vi "Is Command or Response.vi"(8 "error in (no error)":errorcluster, 11 "Command/Response Refnum in":T1 format="%.0x") -> (0 "error out":errorcluster, 2 "Is Command?":bool, 3 "Command/Response out":string)   [LabVIEW 2018, in "Instrument Addon Scripting API.lvlib"]
uses:
  Instrument Addon Scripting API.lvlib
  <vilib>/NI Veristand/Custom Device API/Custom Device Item Ref.ctl
  Addon/Addon Shared/SubVIs/Constants.vi
  Addon/Addon Shared/Instrument Addon Shared.lvlib
  <vilib>/NI VeriStand/Custom Device API/Custom Device API.lvlib
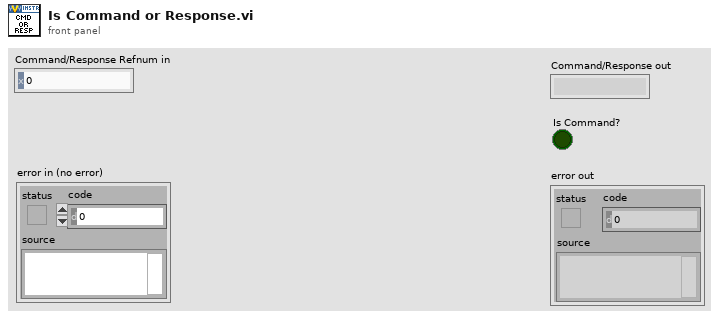
[diagram p1: front panel]
types:
  T1 = typedef "Custom Device API.lvlib/Custom Device Item Ref.ctl" = u64
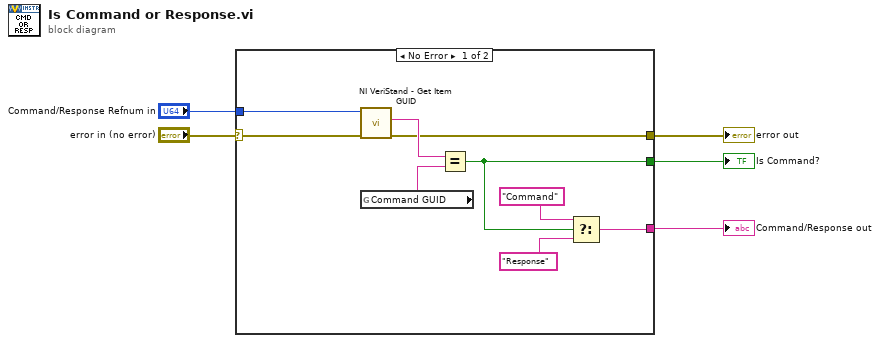
[diagram p0: block diagram]
diagram:
  n1 = case shown="No Error" "error in (no error)" {
    selector: "error in (no error)" -> [w6 w15]
    tunnel: [w14 _] -> w5
    tunnel: [w11 w15] -> w4
    tunnel: "Command/Response Refnum in" -> [w8 _]
    tunnel: [w7 _] -> w2
    frame No Error {
      n2 = call <vilib>:"NI VeriStand - Get Item GUID.vi"("error in (no error)"=w6, "Item Ref in"=w8) -> ("error out"=w11:errorcluster, "GUID"=w12:string)  [unwired: 7 in, 1 out]
      n3 = global read "Constants.vi" "Command GUID"() -> (w13:string)
      n4 = Equal?(x=w12, y=w13) -> (x = y?=w14:bool)
      n5 = Select(t="Command", s=w14, f="Response") -> (s? t:f=w7:string)
    }
    frame Error {
    }
  }
  "error out" <- w4
  "Command/Response out" <- w2
  "Is Command?" <- w5
